vi "1726 Turn by Angle.vi"(0 "RobotDriveDevRef in":T2, 1 "Target Angle":dbl, 2 "Tuning Parametres":T1) -> (7 "RobotDriveDevRef out":T2, 9 "Is Finished?":bool, 10 "Is Timedout?":bool)   [LabVIEW 2017]
uses:
  <vilib>/Rock Robotics/WPI/RobotDrive/WPI_RobotDriveDevRef.ctl
  <vilib>/Rock Robotics/WPI/MotorControl/WPI_MotorControlDeviceRef.ctl
  <vilib>/Rock Robotics/WPI/MotorControl/WPI_MotorControlType.ctl
  <vilib>/Rock Robotics/SystemInterfaces/DIO/FPGA_DIOPWMChannel.ctl
  <vilib>/Rock Robotics/WPI/PWM/WPI_PWMDeadband.ctl
  <vilib>/Rock Robotics/SystemInterfaces/DIO/FPGA_DIOChannel.ctl
  Team Code/Robot Global Data.vi
  <vilib>/addons/control/pid/pid.llb/PID Advanced (DBL).vi
  <vilib>/Rock Robotics/WPI/RobotDrive/WPI_RobotDriveArcadeDrive_Standard(NoSaturation).vi
  <vilib>/addons/control/pid/NI_PID_pid.lvlib
panel:
  in  "Timeout (ms)":u32
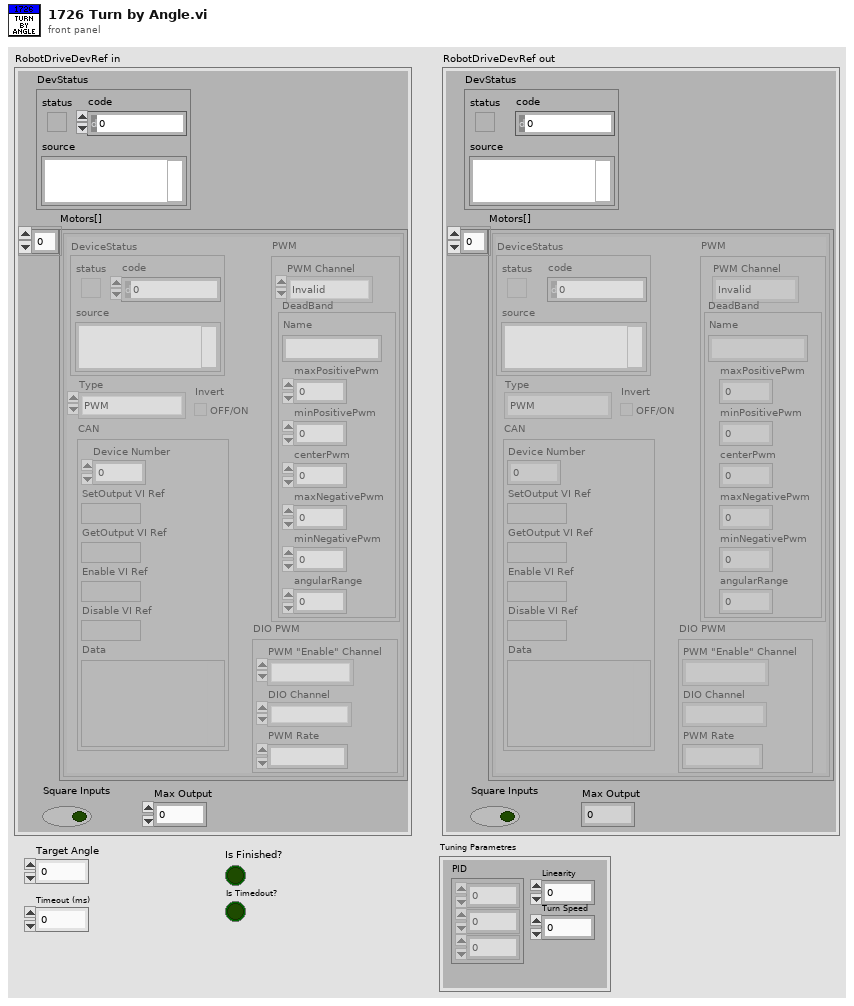
[diagram p1: front panel]
types:
  T1 = cluster{"PID":dbl[], "Linearity":dbl, "Turn Speed":dbl}
  T2 = typedef "WPI_RobotDriveDevRef.ctl" = cluster{"DevStatus":errorcluster, "Motors[]":T3[], "Square Inputs":bool, "Max Output":dbl}
  T3 = typedef "WPI_MotorControlDeviceRef.ctl" = cluster{"DeviceStatus":errorcluster, "Type":T4, "PWM":cluster{"PWM Channel":T5, "DeadBand":T6}, "CAN":cluster{"Device Number":u8, "SetOutput VI Ref":variant, "GetOutput VI Ref":variant, "Enable VI Ref":variant, "Disable VI Ref":variant, "Data":variant}, "Invert":bool, "DIO PWM":cluster{"PWM \"Enable\" Channel":T5, "DIOChannel":T7, "PWM Rate":dbl}}
  T4 = typedef "WPI_MotorControlType.ctl" = enum16{"PWM", "CAN", "DIO PWM"}
  T5 = typedef "FPGA_DIOPWMChannel.ctl" = enum8{"PWM 0", "PWM 1", "PWM 2", "PWM 3", "PWM 4", "PWM 5", "PWM 6", "PWM 7", "PWM 8", "PWM 9", "PWM MXP 0", "PWM MXP 1", "PWM MXP 2", "PWM MXP 3", "PWM MXP 4", "PWM MXP 5", "PWM MXP 6", "PWM MXP 7", "PWM MXP 8", "PWM MXP 9", "Invalid"}
  T6 = typedef "WPI_PWMDeadband.ctl" = cluster{"Name":string, "maxPositivePwm":i32, "minPositivePwm":i32, "centerPwm":i32, "maxNegativePwm":i32, "minNegativePwm":i32, "angularRange":u16}
  T7 = typedef "FPGA_DIOChannel.ctl" = enum8{"DIO 0", "DIO 1", "DIO 2", "DIO 3", "DIO 4", "DIO 5", "DIO 6", "DIO 7", "DIO 8", "DIO 9", "DIO MXP 0", "DIO MXP 1", "DIO MXP 2", "DIO MXP 3", "DIO MXP 4", "DIO MXP 5", "DIO MXP 6", "DIO MXP 7", "DIO MXP 8", "DIO MXP 9", "DIO MXP 10", "DIO MXP 11", "DIO MXP 12", "DIO MXP 13", "DIO MXP 14", "DIO MXP 15", "SPI Port CS1", "SPI Port CS2", "SPI Port CS3", "SPI Port MISO", "SPI Port MOSI", "Invalid"}
  T8 = cluster{"PID[0]":dbl, "PID[1]":dbl, "PID[2]":dbl}
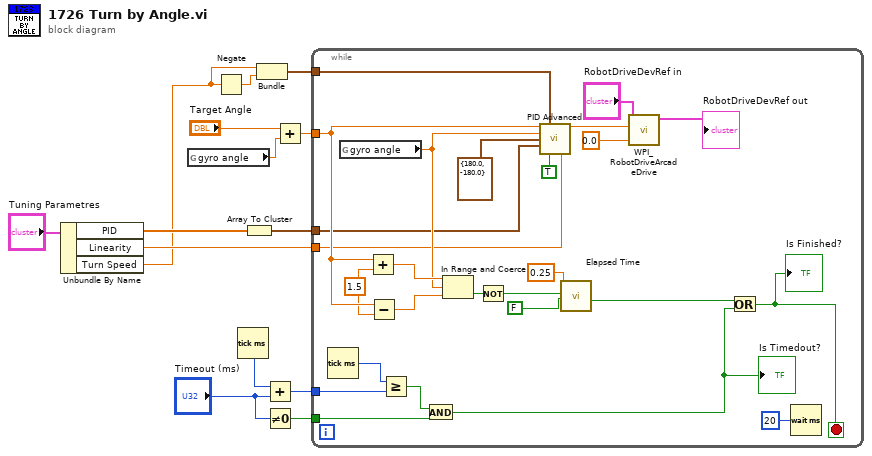
[diagram p0: block diagram]
diagram:
  n1 = Unbundle By Name("Tuning Parametres") -> ("PID"=w4:dbl[], "Linearity"=w2:dbl, "Turn Speed"=w1:dbl)
  n2 = global read "Robot Global Data.vi" "gyro angle"() -> (w13:dbl)
  n3 = Negate(x=w1) -> (-x=w7:dbl)
  n4 = Tick Count (ms)() -> (millisecond timer value=w11:u32)
  n5 = Array To Cluster(array=w4) -> (cluster=w3:T8)
  n6 = Bundle("Turn Speed"=w1, w7) -> (w6:cluster{"Turn Speed":dbl, dbl})  [unwired: 1 in]
  n7 = Add(x=w11, y="Timeout (ms)") -> (x+y=w9:u32)
  n8 = Not Equal To 0?(x="Timeout (ms)") -> (x != 0?=w8:bool)
  n9 = Add(x="Target Angle", y=w13) -> (x+y=w12:dbl)
  n10 = while {
    tunnel: w12 -> [w26]
    tunnel: w9 -> [w22]
    tunnel: w8 -> [w21]
    tunnel: w6 -> [w17]
    tunnel: w3 -> [w16]
    tunnel: w2 -> [w15]
    stop <- w19 stop-if-true
    w25 = 1.5 ("y")
    n11 = Tick Count (ms)() -> (millisecond timer value=w24:u32)
    n12 = global read "Robot Global Data.vi" "gyro angle"() -> (w27:dbl)
    n13 = Add(x=w26, y=w25) -> (x+y=w34:dbl)
    n14 = Subtract(x=w26, y=w25) -> (x-y=w33:dbl)
    n15 = Greater Or Equal?(x=w24, y=w22) -> (x >= y?=w23:bool)
    n16 = And(x=w23, y=w21) -> (x .and. y?=w18:bool)
    "Is Timedout?" <- w18
    n17 = In Range and Coerce(upper limit=w34, x=w27, lower limit=w33) -> (In Range?=w29:bool)  [unwired: 1 out]
    n18 = Not(x=w29) -> (.not. x?=w30:bool)
    n19 = call-poly <vilib>:"PID Advanced.vi"("setpoint"=w26, "output range"=w17, "process variable"=w27, "setpoint range"=cluster{"setpoint high":dbl, "setpoint low":dbl} {"setpoint high"=180.0, "setpoint low"=-180.0}, "PID gains"=w16, "reinitialize? (F)"=TRUE, "linearity"=w15) -> ("output"=w37:dbl)  [unwired: 7 in, 1 out]
    n20 = call "Elapsed Time"("Time Target (s)"=0.25, "Reset"=w30, "Auto Reset"=FALSE) -> ("Time has Elapsed"=w20:bool)  [unwired: 9 in, 7 out]
    n21 = call-poly <vilib>:"WPI_RobotDriveArcadeDrive.vi"("Y axis value"=0.0, "X axis value"=w37, "RobotDriveDevRef"="RobotDriveDevRef in") -> ("RobotDriveDevRef"=→"RobotDriveDevRef out":T2)  [unwired: 1 in, 7 out]
    n22 = Or(x=w20, y=w18) -> (x .or. y?=w19:bool)
    "Is Finished?" <- w19
    n23 = Wait (ms)(milliseconds to wait=u32 20 ("millisecond timer value")) -> ()  [unwired: 1 out]
  }
